vi "GetFlatSequences.vi"(6 "error in":errorcluster, 9 "Diagram in":refnum<class "Diagram.lvclass">) -> (0 "error out":errorcluster, 3 "Diagram out":refnum<class "Diagram.lvclass">, 4 "flat sequences":i32[](array[numeric]))   [LabVIEW 2014, in "Diagram.lvclass"]
uses:
  Diagram.lvclass
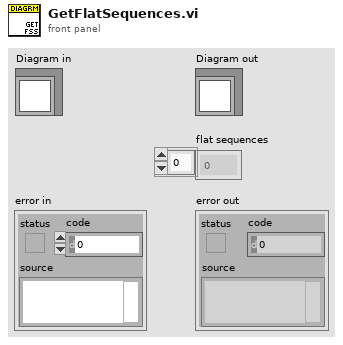
[diagram p1: front panel]
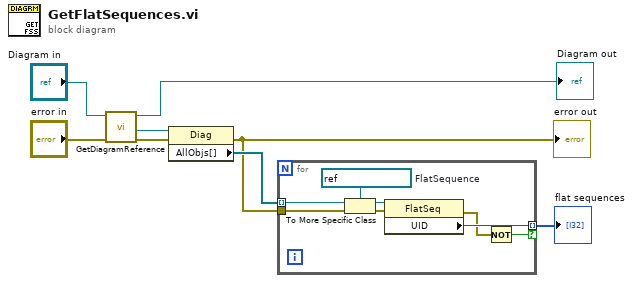
[diagram p0: block diagram]
diagram:
  n1 = call "GetDiagramReference.vi"("error in"="error in", "Diagram in"="Diagram in") -> ("error out"=w6:errorcluster, "reference out"=w5:refnum<vi>, "Diagram out"=→"Diagram out":refnum<class "Diagram.lvclass">)  [unwired: 5 in]
  n2 = property class="Diag"(reference=w5, error in=w6) -> (error out=w2:errorcluster, "AllObjs[]"=w4:refnum<vi>[])  [unwired: 1 out]
  "error out" <- w2
  n3 = for {
    tunnel: w4 -> [w16] mode=indexing
    tunnel: w2 -> [w15]
    tunnel: [w11] -> w3 mode=indexing if=w9
    w14 = refnum<vi> refnum  # FlatSequence
    n4 = To More Specific Class(target class=w14, reference=w16, error in=w15) -> (specific class reference=w13:refnum<vi>, error out=w12:errorcluster)
    n5 = property class="FlatSeq"(reference=w13, error in=w12) -> (error out=w10:errorcluster, "UID"=w11:i32)  [unwired: 1 out]
    n6 = Not(x=w10) -> (.not. x?=w9:bool)
  }
  "flat sequences" <- w3
